vi "array -- 2D mean .vi"(11 "pond":cdb[][](array[numeric])) -> (1 "mean row":dbl, 2 "mean col":dbl)   [LabVIEW 2015]
uses:
  <vilib>/Analysis/baseanly.llb/Real A x B.vi
  <vilib>/Analysis/baseanly.llb/Mean (DBL).vi
  <vilib>/Analysis/NI_AALBase.lvlib
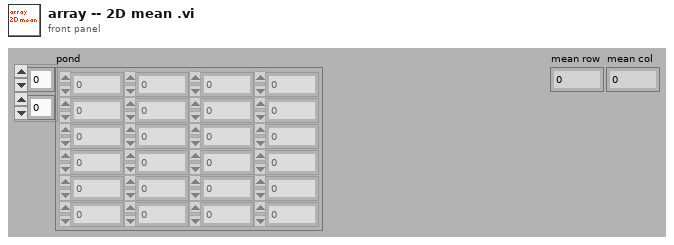
[diagram p1: front panel]
types:
  T1 = typedef "NI_Matrix.lvlib/RealMatrix.ctl" = dbl[][]
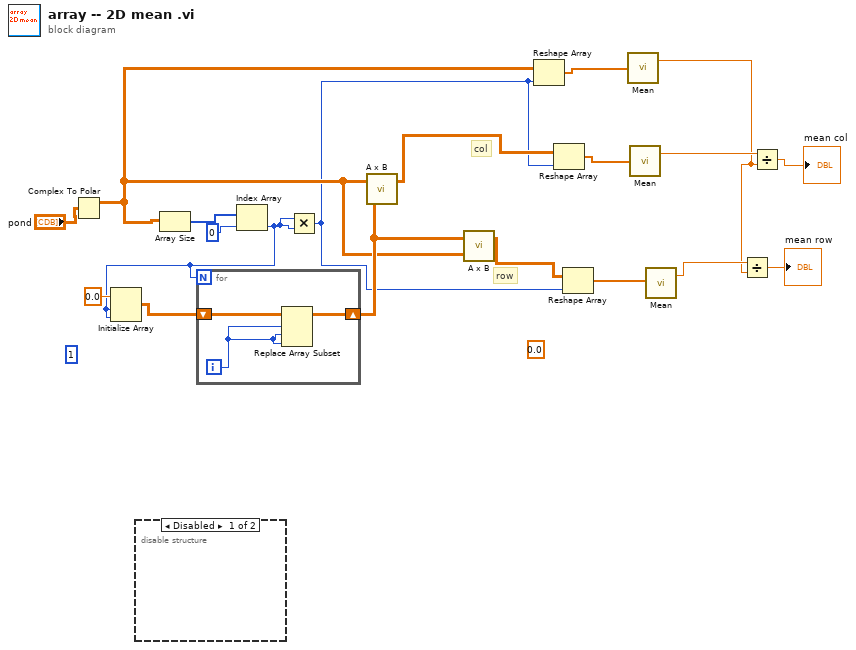
[diagram p0: block diagram]
diagram:
  (unwired) 0.0 ("element")
  (unwired) 1 ("index")
  # "row"
  # "col"
  n1 = Complex To Polar(r * e^(i*theta)="pond") -> (r=w7:dbl[][])  [unwired: 1 out]
  n2 = disable-structure shown="Disabled" {
    frame Disabled {
    }
    frame Enabled {
    }
  }
  n3 = Array Size(array=w7) -> (size(s)=w19:i32[])
  n4 = Index Array(array=w19, index=0) -> (element=w14:i32)
  n5 = Initialize Array(0.0 ("element"), w14, w14) -> (w16:dbl[][])
  n6 = for {
    N: w14 -> [_]
    shift-right: [w21] -> w15
    shift-left: w16 -> [w22]
    i -> [w20]
    n7 = Replace Array Subset(array=w22, new element=w20, index (row)=w20, index (col)=w20) -> (w21:T1)
  }
  n8 = Multiply(x=w14, y=w14) -> (x*y=w1:i32)
  n9 = call-poly <vilib>:"A x B.vi"("B"=w15, "A"=w7) -> ("A x B"=w13:T1)  [unwired: 1 out]
  n10 = call-poly <vilib>:"A x B.vi"("B"=w7, "A"=w15) -> ("A x B"=w12:T1)  [unwired: 1 out]
  n11 = Reshape Array(w7, w1) -> (w10:dbl[])
  n12 = Reshape Array(w13, w1) -> (w9:dbl[])
  n13 = Reshape Array(w12, w1) -> (w11:dbl[])
  n14 = call-poly <vilib>:"Mean.vi"("X"=w10) -> ("mean"=w4:dbl)  [unwired: 1 out]
  n15 = call-poly <vilib>:"Mean.vi"("X"=w9) -> ("mean"=w6:dbl)  [unwired: 1 out]
  n16 = call-poly <vilib>:"Mean.vi"("X"=w11) -> ("mean"=w5:dbl)  [unwired: 1 out]
  n17 = Divide(x=w5, y=w4) -> (x/y=→"mean row":dbl)
  n18 = Divide(x=w6, y=w4) -> (x/y=→"mean col":dbl)
